vi "Gamma Noise Waveform.vi"(6 "sampling info":cluster{"Fs":dbl, "#s":dbl}={"Fs"=1000.0, "#s"=1000.0} {"Fs" format="%.2p"}, 7 "reset signal":bool, 8 "error in (no error)":errorcluster, 10 "seed":i32=-1, 11 "order":i32=1) -> (0 "error out":errorcluster, 3 "signal out":waveform(dbl))   [LabVIEW 2020, in "NI_MABase.lvlib"]
doc: "Generates a pseudorandom pattern of values which are the waiting times to the <B>order</B> number event of a unit mean Poisson process."
uses:
  NI_MABase.lvlib
  NI_AALBase.lvlib
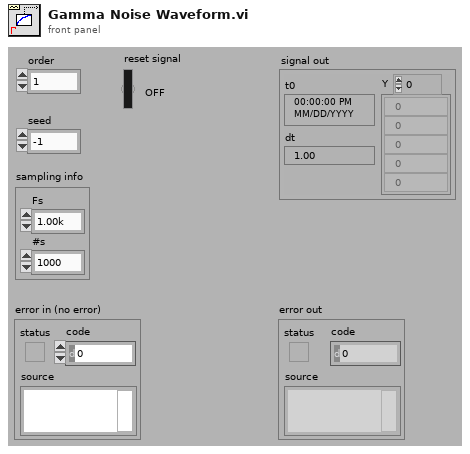
[diagram p1: front panel]
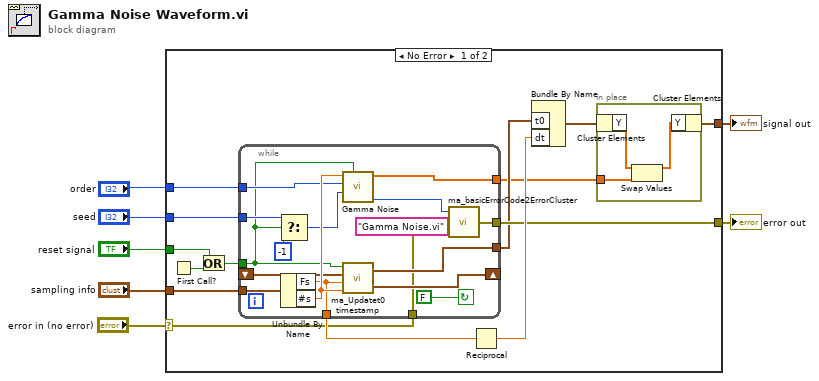
[diagram p0: block diagram]
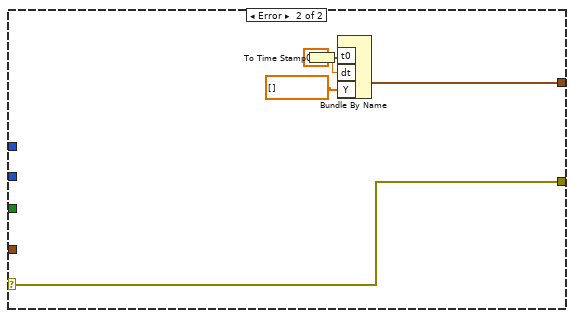
[diagram p2: hidden frame]
diagram:
  n1 = case shown="No Error" "error in (no error)" {
    selector: "error in (no error)" -> [w15 w46]
    tunnel: [w20 w46] -> w7
    tunnel: "sampling info" -> [w19 _]
    tunnel: "order" -> [w17 _]
    tunnel: "seed" -> [w16 _]
    tunnel: [w8 w43] -> w2
    tunnel: "reset signal" -> [w11 _]
    frame No Error {
      n2 = First Call?() -> (First Call?: T/F=w13:bool)
      n3 = Or(x=w11, y=w13) -> (x .or. y?=w12:bool)
      n4 = while {
        tunnel: w15 -> [w29]
        tunnel: w12 -> [w25]
        tunnel: w16 -> [w28]
        tunnel: w17 -> [w30]
        tunnel: [w33] -> w18
        tunnel: w19 -> [w34]
        tunnel: [w36] -> w9
        tunnel: [w37] -> w14
        shift-left: _ -> [w39]
        shift-right: [w38] -> _
        tunnel: [w40] -> w20
        stop <- FALSE continue-if-true
        n5 = Select(t=w28, s=w25, f=-1) -> (s? t:f=w27:i32)
        n6 = Unbundle By Name(w34) -> ("Fs"=w33:dbl, "#s"=w41:dbl)
        n7 = call "Gamma Noise.vi"("initialize?"=w25, "seed"=w27, "order"=w30, "samples"=w41) -> ("error"=w32:i32, "gamma noise"=w36:dbl[])  [unwired: 6 in]
        n8 = call "ma_Updatet0 timestamp.vi"("samples"=w41, "sampling rate (S/s)"=w33, "tf previous"=w39, "Reset Generation"=w25) -> ("tf new"=w38:timestamp, "t0"=w37:timestamp)
        n9 = call "ma_basicErrorCode2ErrorCluster.vi"("error in (no error)"=w29, "subVI name"="Gamma Noise.vi" ("subVI Name"), "Error Code"=w32) -> ("error out"=w40:errorcluster)
      }
      n10 = Reciprocal(x=w18) -> (1/x=w21:dbl)
      n11 = Bundle By Name("t0"=w14, "dt"=w21) -> (w10:waveform(dbl))  [unwired: 1 out]
      n12 = in-place {
        in-place-border: w9 -> [w22]
        n13 = in-place-cluster #1(w10) -> ("Y"=w24:dbl[])
        n14 = Swap Values(12:w24, 14:w22) -> (1:w23:dbl[])  [unwired: 1 in, 1 out]
        n15 = in-place-cluster #1("Y"=w23) -> (w8:waveform(dbl))
      }
    }
    frame Error {
      w45 = 0.0 ("t0")
      n16 = To Time Stamp(1:w45) -> (0:w42:timestamp)
      n17 = Bundle By Name("t0"=w42, "dt"=w45, "Y"=dbl[] []) -> (w43:waveform(dbl))  [unwired: 1 out]
    }
  }
  "error out" <- w7
  "signal out" <- w2
